vi "Get_Open_VIs.vi"() -> ()   [LabVIEW 2010]
uses:
  Module.ctl
panel:
  in  "Module":string
  out "Module (OUT)":T1
  in  "Module (IN)":T1
  in  "Start/Stop?":enum16{"Start", "Stop"}(ring)
  out "error out":errorcluster
  in  "error in (no error)":errorcluster
  out "All VIs In Memory":string[](array[string])
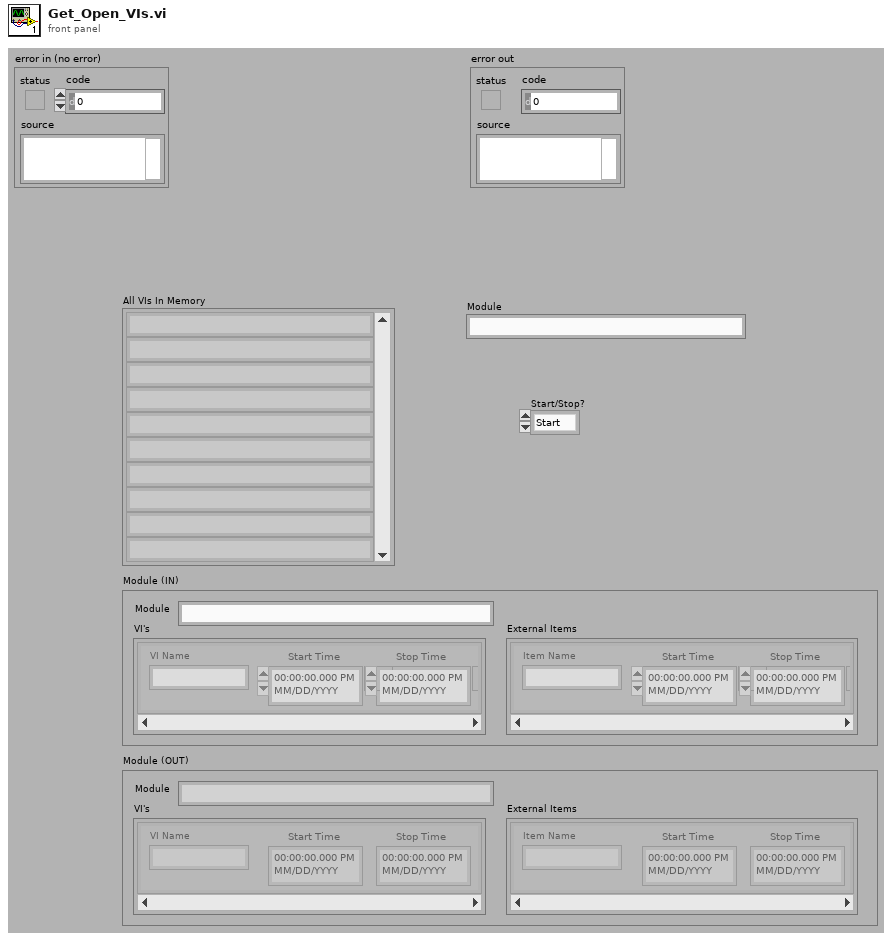
[diagram p1: front panel]
types:
  T1 = typedef "Module.ctl" = cluster{"VI's":cluster{"VI Name":string, "Start Time":timestamp, "Stop Time":timestamp}[], "External Items":cluster{"Item Name":string, "Start Time":timestamp, "Stop Time":timestamp}[], "Module":string}
  T2 = cluster{"Item Name":string, "Start Time":timestamp, "Stop Time":timestamp}[]
  T3 = cluster{"VI Name":string, "Start Time":timestamp, "Stop Time":timestamp}[]
  T4 = cluster{"VI Name":string, "Start Time":timestamp, "Stop Time":timestamp}
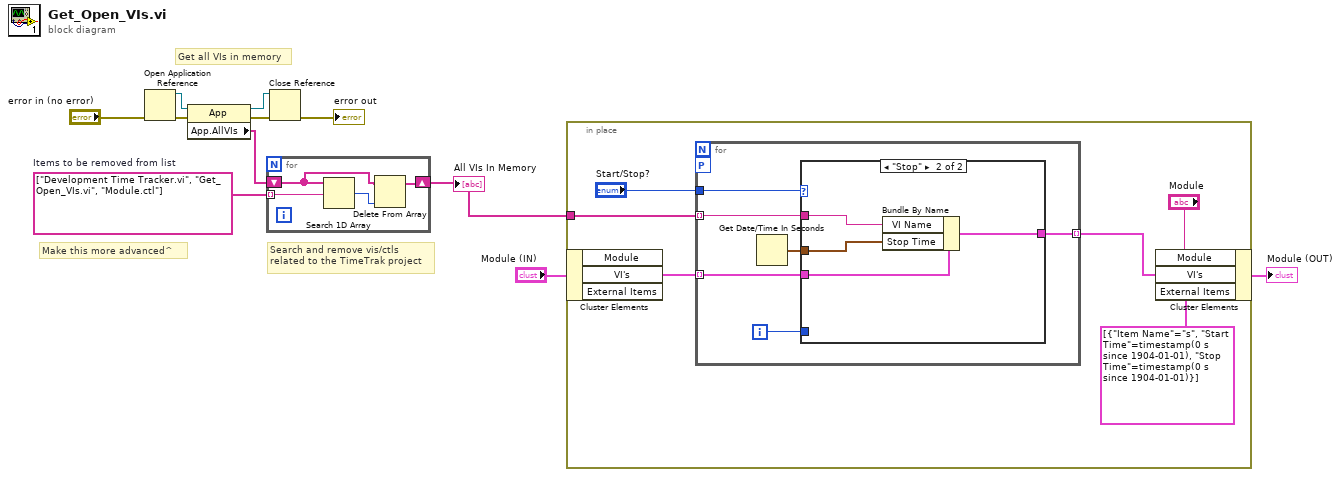
[diagram p0: block diagram]
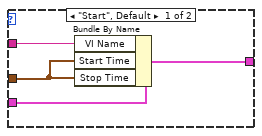
[diagram p2: hidden frame]
diagram:
  w6 = string[] ["Development Time Tracker.vi", "Get_Open_VIs.vi", "Module.ctl"]  # Items to be removed from list
  # "Get all VIs in memory"
  # "Search and remove vis/ctls\nrelated to the TimeTrak project"
  # "Make this more advanced^"
  n1 = Open Application Reference(8:"error in (no error)") -> (0:w10:errorcluster, 3:w5:refnum<vi>)  [unwired: 3 in]
  n2 = property class="App"(reference=w5, error in=w10) -> (reference out=w4:refnum<vi>, error out=w11:errorcluster, "App.AllVIs"=w7:string[])
  n3 = for {
    tunnel: w6 -> [w15] mode=indexing
    shift-right: [w13] -> w2
    shift-left: w7 -> [w14]
    n4 = Search 1D Array(1D array=w14, element=w15) -> (index of element=w12:i32)  [unwired: 1 in]
    n5 = Delete From Array(array=w14, index=w12) -> (array with subset deleted=w13:string[])  [unwired: 1 in, 1 out]
  }
  "All VIs In Memory" <- w2
  n6 = Close Reference(reference=w4, error in (no error)=w11) -> (error out=→"error out":errorcluster)
  n7 = in-place {
    in-place-border: w2 -> [w19]
    n8 = in-place-cluster #1("Module (IN)") -> ("VI's"=w16:T3)  [unwired: 2 out]
    n9 = for {
      tunnel: w19 -> [w27] mode=indexing
      tunnel: w16 -> [w23] mode=indexing
      tunnel: "Start/Stop?" -> [w26]
      tunnel: [w24] -> w18 mode=indexing
      workers-P: _ -> [_]
      i -> [w22]
      n10 = Get Date/Time In Seconds() -> (seconds since 1Jan1904=w25:timestamp)
      n11 = case shown="\"Stop\"" w26 {
        tunnel: w27 -> [w31 w35]
        tunnel: w25 -> [w30 w34]
        tunnel: [w28 w33] -> w24
        tunnel: w23 -> [w29 w32]
        tunnel: w22 -> [_ _]
        frame "Start", Default {
          n12 = Bundle By Name(cluster=w29, "VI Name"=w31, "Start Time"=w30, "Stop Time"=w30) -> (w28:T4)
        }
        frame "Stop" {
          n13 = Bundle By Name(cluster=w32, "VI Name"=w35, "Stop Time"=w34) -> (w33:T4)
        }
      }
    }
    n14 = in-place-cluster #1("Module"="Module", "VI's"=w18, "External Items"=T2 [{"Item Name"="s", "Start Time"=timestamp(0 s since 1904-01-01), "Stop Time"=timestamp(0 s since 1904-01-01)}]) -> (→"Module (OUT)":T1)
  }
